vi "Image_Burst_Framerate.vi"(8 "Checkbox":bool, 11 "input cluster":T1={"L16 Linear Actuator"="", "XE 1000 Pump"="", "Camera1"="", "Camera2"="", "Camera1_IMG"=refnum, "Camera2_IMG"=refnum, "Img_Capt"=FALSE, "Actuator"=FALSE, "Pump"=FALSE, "Cam 1"=FALSE, "Cam 2"=FALSE, "Empty_Refill"=FALSE, "Crop"=FALSE, "Period"=10, "Light intensity"=100, "Exposure Time"=1000.0, "Sample Name"="Test Sample", "Operator"="MRJ", "Calibration 1"=path "C:/Users/au540322/Desktop/IHS_Project/images/Debris/Debris_0/Debris_0_2019_06_01-23-32-49-686.PNG", "Calibration 2"=path "C:/Users/au540322/Desktop/IHS_Project/images/Debris/Debris_0/Debris_0_2019_06_01-23-32-49-686.PNG", "Framerate"=100, "Timeout Sample"=200, "Sample Frequency"=200, "Notes/Description"="", "Cam 1 queue"=refnum, "Cam 2 queue"=refnum, "Sample size threshold"=500, "Empty start"=1, "Command"="", "Cam 1 - save queue"=refnum, "Cam 2 - save queue"=refnum, "Calibration Image 1"=refnum, "Calibration Image 2"=refnum, "Original Image 1"=refnum, "Original Image 2"=refnum, "Processing Image 1"=refnum, "Processing Image 2"=refnum, "Object Image 1"=refnum, "Object Image 2"=refnum} {"Empty start" min=1; "Sample size threshold" min=1; "Sample Frequency" min=1; "Framerate" min=1; "Light intensity" scale=0.0..100.0}) -> (3 "output cluster":T1={"L16 Linear Actuator"="", "XE 1000 Pump"="", "Camera1"="", "Camera2"="", "Camera1_IMG"=refnum, "Camera2_IMG"=refnum, "Img_Capt"=FALSE, "Actuator"=FALSE, "Pump"=FALSE, "Cam 1"=FALSE, "Cam 2"=FALSE, "Empty_Refill"=FALSE, "Crop"=FALSE, "Period"=10, "Light intensity"=100, "Exposure Time"=1000.0, "Sample Name"="Test Sample", "Operator"="MRJ", "Calibration 1"=path "C:/Users/au540322/Desktop/IHS_Project/images/Debris/Debris_0/Debris_0_2019_06_01-23-32-49-686.PNG", "Calibration 2"=path "C:/Users/au540322/Desktop/IHS_Project/images/Debris/Debris_0/Debris_0_2019_06_01-23-32-49-686.PNG", "Framerate"=100, "Timeout Sample"=200, "Sample Frequency"=200, "Notes/Description"="", "Cam 1 queue"=refnum, "Cam 2 queue"=refnum, "Sample size threshold"=500, "Empty start"=1, "Command"="", "Cam 1 - save queue"=refnum, "Cam 2 - save queue"=refnum, "Calibration Image 1"=refnum, "Calibration Image 2"=refnum, "Original Image 1"=refnum, "Original Image 2"=refnum, "Processing Image 1"=refnum, "Processing Image 2"=refnum, "Object Image 1"=refnum, "Object Image 2"=refnum} {"Empty start" min=1; "Sample size threshold" min=1; "Sample Frequency" min=1; "Framerate" min=1; "Light intensity" scale=0.0..100.0})   [LabVIEW 2019]
uses:
  controls/Data.ctl
  <vilib>/userdefined/High Color/IMAQdx.ctl
  <vilib>/vision/Image Controls.llb/IMAQ Image.ctl
  <resource>/objmgr/imaqdx.rc
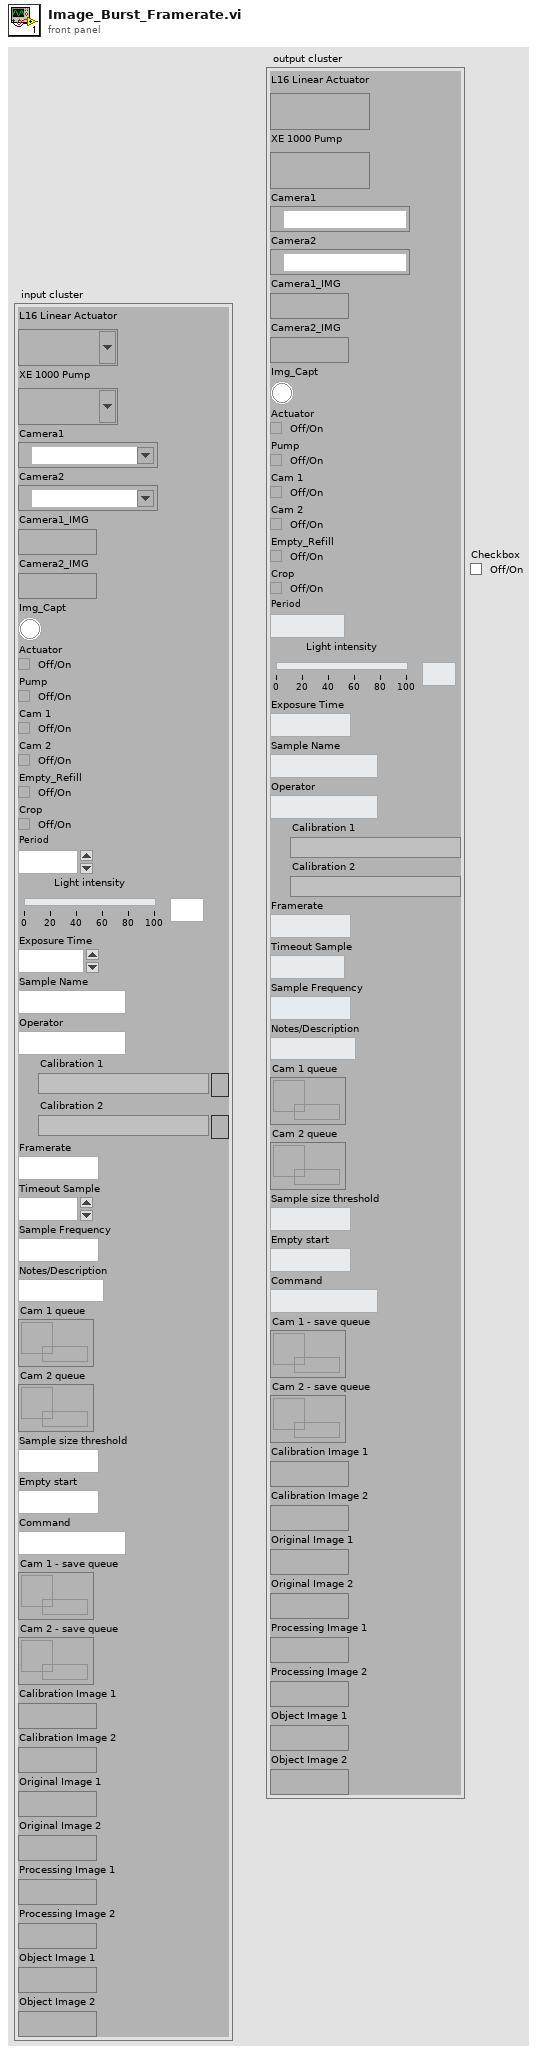
[diagram p1: front panel]
types:
  T1 = typedef "Data.ctl" = cluster{"L16 Linear Actuator":refnum<visa-resource-name>, "XE 1000 Pump":refnum<visa-resource-name>, "Camera1":T2, "Camera2":T2, "Camera1_IMG":T3, "Camera2_IMG":T3, "Img_Capt":bool, "Actuator":bool, "Pump":bool, "Cam 1":bool, "Cam 2":bool, "Empty_Refill":bool, "Crop":bool, "Period":i64, "Light intensity":i32, "Exposure Time":dbl, "Sample Name":string, "Operator":string, "Calibration 1":path, "Calibration 2":path, "Framerate":i32, "Timeout Sample":i32, "Sample Frequency":i32, "Notes/Description":string, "Cam 1 queue":refnum<queue>, "Cam 2 queue":refnum<queue>, "Sample size threshold":i32, "Empty start":u32, "Command":string, "Cam 1 - save queue":refnum<queue>, "Cam 2 - save queue":refnum<queue>, "Calibration Image 1":T3, "Calibration Image 2":T3, "Original Image 1":T3, "Original Image 2":T3, "Processing Image 1":T3, "Processing Image 2":T3, "Object Image 1":T3, "Object Image 2":T3}
  T2 = typedef "IMAQdx.ctl" = refnum<k21>
  T3 = typedef "IMAQ Image.ctl" = refnum<image>
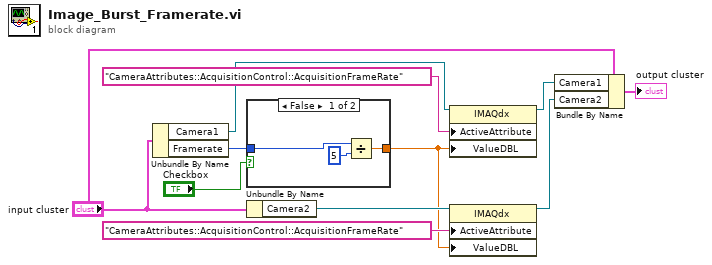
[diagram p0: block diagram]
diagram:
  n1 = Unbundle By Name("input cluster") -> ("Camera1"=w11:T2, "Framerate"=w3:i32)
  n2 = case shown="False" "Checkbox" {
    tunnel: w3 -> [w14 w15]
    tunnel: [w13 w15] -> w2
    frame False {
      n3 = Divide(x=w14, y=5) -> (x/y=w13:dbl)
    }
    frame True {
    }
  }
  n4 = Unbundle By Name("input cluster") -> ("Camera2"=w7:T2)
  n5 = property class="IMAQdx"(reference=w11, "ActiveAttribute"="CameraAttributes::AcquisitionControl::AcquisitionFrameRate", "ValueDBL"=w2) -> (reference out=w9:T2)  [unwired: 1 in, 1 out]
  n6 = property class="IMAQdx"(reference=w7, "ActiveAttribute"="CameraAttributes::AcquisitionControl::AcquisitionFrameRate", "ValueDBL"=w2) -> (reference out=w5:T2)  [unwired: 1 in, 1 out]
  n7 = Bundle By Name(cluster="input cluster", "Camera1"=w9, "Camera2"=w5) -> (→"output cluster":T1)
